vi "LabVIEW_Example.vi"() -> ()   [LabVIEW 2016]
panel:
  in  "stop":bool
  in  "Tab Control":enum32{"Navigation", "Interface", "About"}(tab)
  out "MoveSignal":bool caption="Moving"
  out "Connected":bool=TRUE
  out "EotrightDetected1":bool caption="Status Eot FWD"
  out "EotLeftDetected1":bool caption="Status Eot BWD"
  out "move out":bool=TRUE caption="Move"
  out "in target range1":bool
  in  "Reset Error":bool
  out "Error":bool
  out "Error Message":string
  in  "Axis Tab Control":enum32{"Operation", "Settings"}(tab)
  out "R [Ohm]":dbl
  out "C [nF]":dbl
  in  "Single Step\nLeft":bool caption="Open Loop Funktions"
  in  "Single Step\nRight":bool caption="Step(s)"
  in  "Continuous Forward 2":bool caption="Continuous\nForward"
  in  "Endless Left":bool caption="Continuous\nBackward"
  in  "Amplitude [V]":dbl=45.001 format="%#.3f"
  in  "Frequency [Hz]":dbl=1998.531 format="%#.3f"
  in  "Fixed DC 1":i32 caption="DC Level [mV]"
  in  "Axis 1":bool caption="Closed Loop Functions"
  out "Position":dbl=14701.126 caption="Position [nm]" format="%#_6f"
  out "Reference":dbl=-7597148.0 caption="Reference position [nm]" format="%#_6f"
  out "ReferenceSignal":bool=TRUE
  in  "measureC&R":bool
  in  "Target Position 1":i32 caption="Target position [µm]"
  in  "Move 2":bool
  in  "Positioner":u16(ring)=15 items=["ECGp5050", "ECGt5050", "ECR3030", "ECR4040", "ECR5050", "ECSx3030", "ECSx3040", "ECSx3050", "ECSx3060", "ECSx3070", "ECSx3080", "ECSx5050", "ECSxy5050", "ECSz3030", "ECSz5050", "EOP1", "EOP2", "EOP3"]
  in  "Number of steps":i32=1 caption="Number of Steps"
  in  "stop_on_EoT":bool caption="Stop on end of travel"
  in  "Target Range 1":u32 caption="Target Range [nm]"
  in  "Sensor Settings Tab Control":enum32{"NUM only", "RES only"}(tab)
  in  "auto Reset 1":bool=TRUE caption="Auto Reset"
  in  "Reference Auto Update 1":bool=TRUE caption="Auto update reference"
  in  "Configuration upload":path
  in  "Gound on target":bool
  in  "Sensor power":enum16{"0 dB", "-10 dB", "-15 dB", "-20 dB"}(ring)
  out "LutSN":string
  in  "auto measure C and R":bool
  in  "Disable Sensor":bool
  in  "Motion control threshold [pm]":i32
  in  "Output":bool=TRUE caption="Axis 1"
  out "Output Status":bool=TRUE
  out "status":string
  out "RT Out Tab Control":enum32{"Off", "AquadB", "Trigger"}(tab)
  in  "AqaudB clock 1":i32 caption="AquadB Clock\n[ns], multiple of 40ns"
  in  "AquadB Resolution 1":i32 caption="AquadB\nResolution [nm]"
  in  "Trigger Config":T1
  out "Error 4":bool caption="Error"
  out "Error Message 4":string
  in  "Mode Input":u16(ring) caption="Mode" items=["Trigger (LVDS)"=11, "Trigger (LVTTL)"=10, "Stepper (LVDS)"=9, "Stepper (LVTTL)"=8, "AquadB (LVDS)"=1, "AquadB (LVTTL)"=0, "OFF"=15]
  in  "Loop Mode":u16(ring) caption="Loop mode" items=["closed-loop"=1, "open-loop"=0]
  in  "Steps per pulse":i32 caption="Steps per pulse [Steps]"
  in  "Change per pulse":i32 caption="Change per pulse [u°/nm]"
  in  "Reset Error 4":bool
  in  "Move":bool=TRUE
  in  "Signal mode":enum16{"LVTTL", "LVDS"}(ring)
  in  "RtOutMode":enum16{"Off", "AquadB", "Trigger"}(ring)
  in  "Reboot":bool
  in  "Factory Reset":bool
  in  "Reset Error 8":bool
  out "Error Message 7":string
  in  "device name (set)":string="myAMC300" caption="Set Device Name"
  out "Error 7":bool caption="Error"
  out "Sn":string caption="Serial Number"
  out "ip":string="192.168.1.1" caption="IP Adress"
  out "Firmware Version":string
  out "Mac Adress":string
  out "authorized\nStatus":bool
  out "locked\nStatus":bool
  out "device name":string caption="Device Name"
  out "Device type":string="AMC100/NUM"
  in  "Unlock":bool=TRUE
  out "Features acivated":string[](array[string])
  in  "Lock":bool=TRUE
  in  "grant access":bool=TRUE
  # "Individual Status Flags"
  # "Closed Loop Functions"
  # "(NUM only)"
  # "Diagnostic Tools (AMC300 only)"
  # "( /PRO Version only )"
  # "( /PRO Version only )"
  # "(AMC300 only)"
  # "Real Time Input"
  # "Real Time Output"
  # "Global Parameters"
  # "Axis 1"
  # "Axis 1"
  # "Device Info"
  # "Device Access"
  # "Features activated"
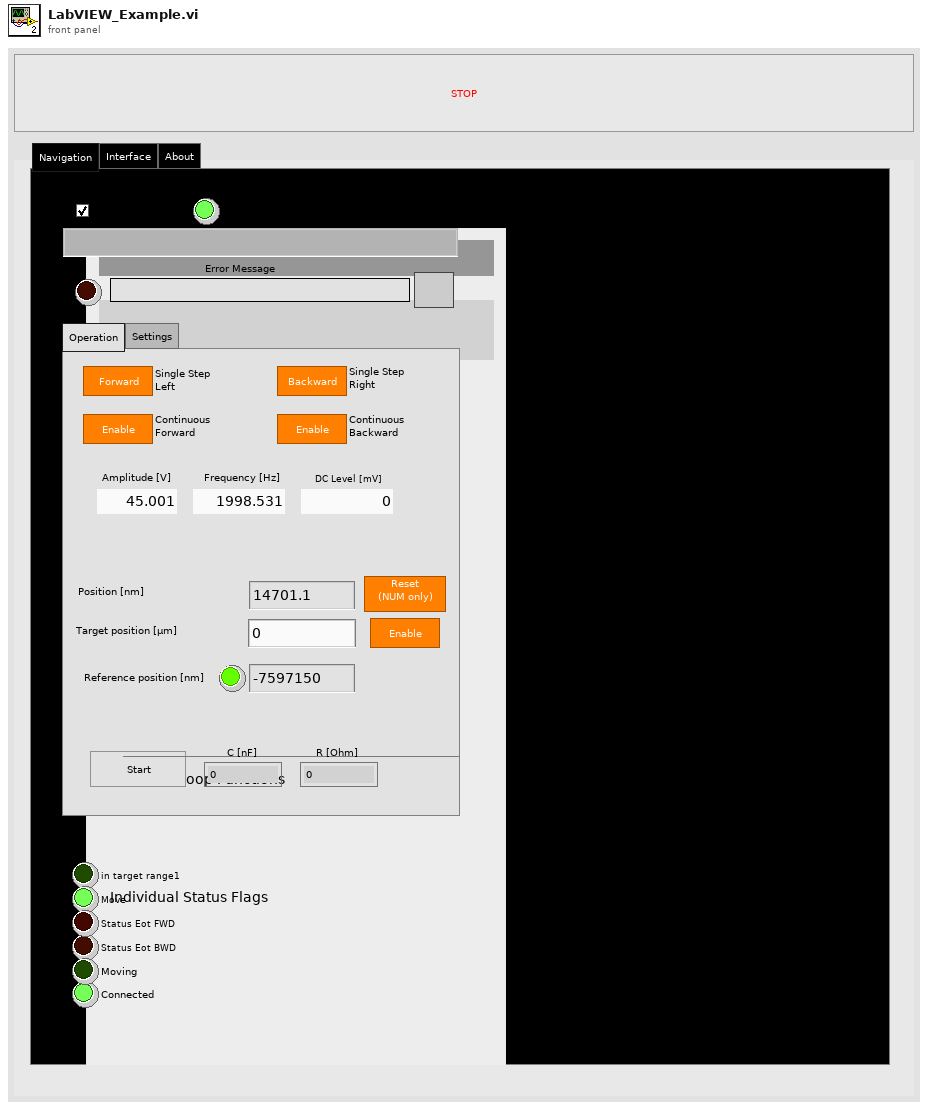
[diagram p1: front panel]
types:
  T1 = cluster{"Position high [nm]":i32, "Position low [nm]":i32, "Trigger polarity":enum16{"Active high", "Active low"}, "Epsilon [nm]":i32}
  T2 = enum8{"Enabled", "Disabled", "Disabled and Grayed Out"}
  T3 = cluster{"serial number":string, "IP address":string, "device type":string, "mac address":string, "device name":string, "firmware version":string}
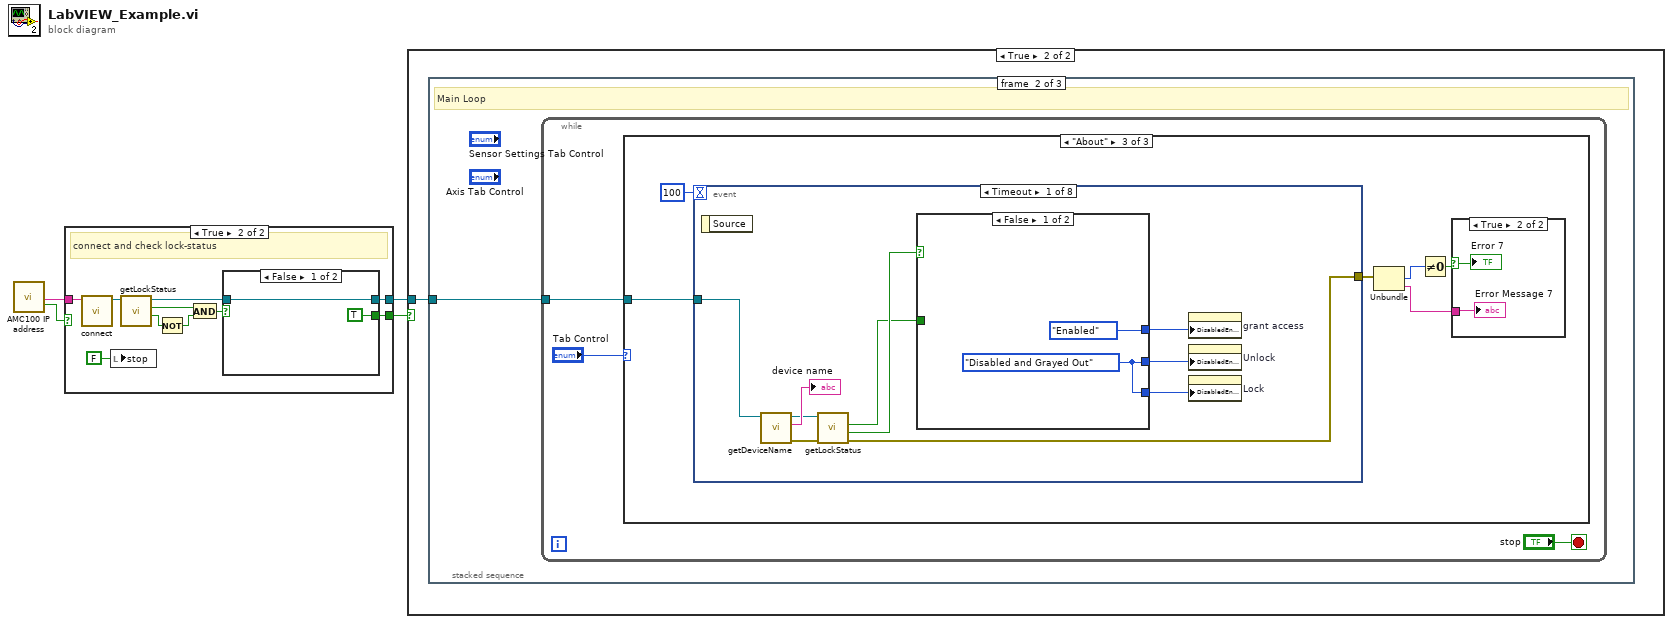
[diagram p0: block diagram]
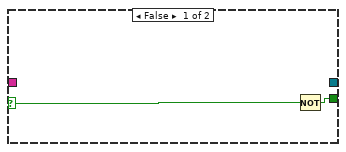
[diagram p2: hidden frame]
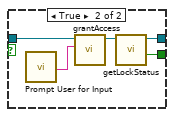
[diagram p3: hidden frame]
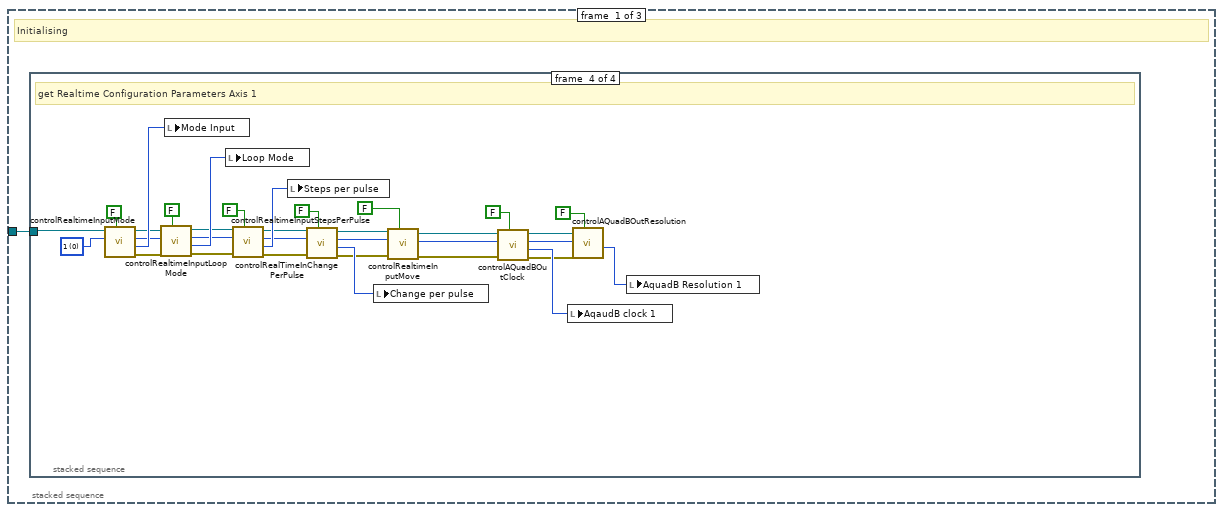
[diagram p5: hidden frame]
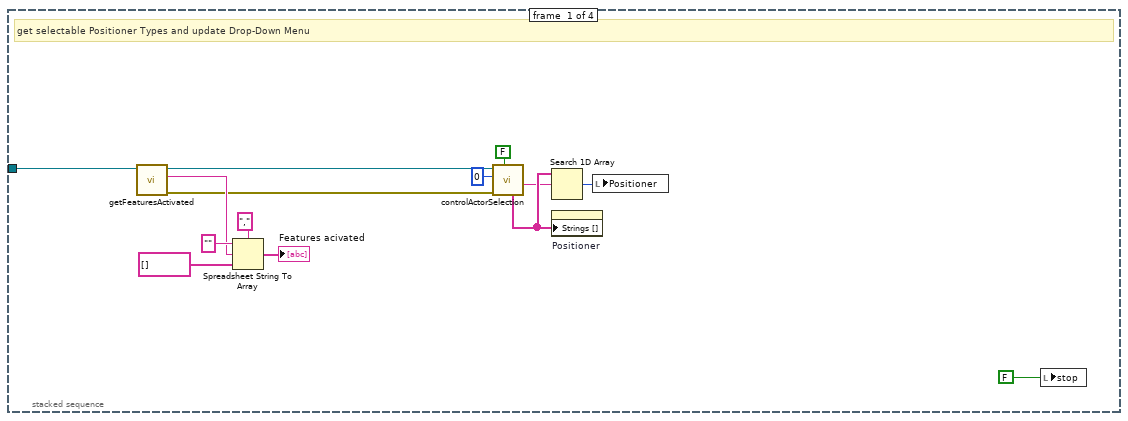
[diagram p6: hidden frame]
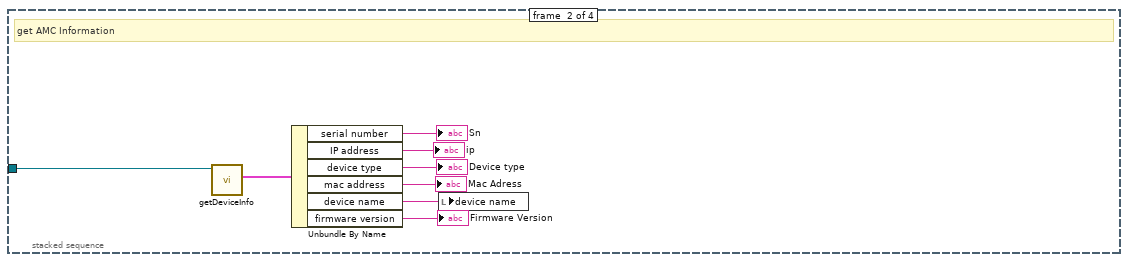
[diagram p7: hidden frame]
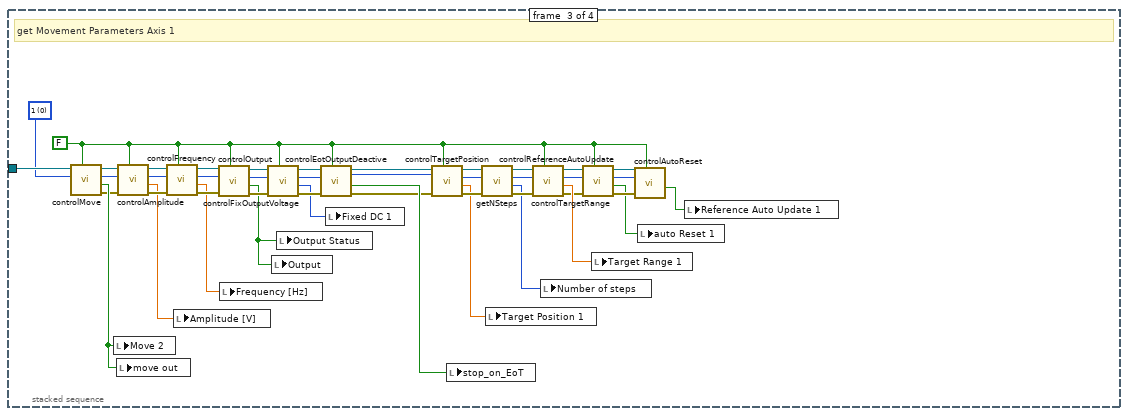
[diagram p8: hidden frame]
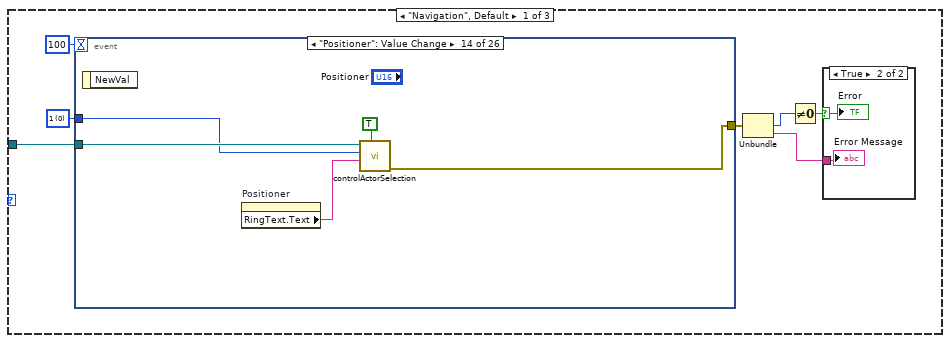
[diagram p9: hidden frame]
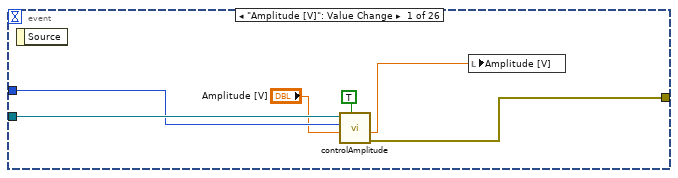
[diagram p11: hidden frame]
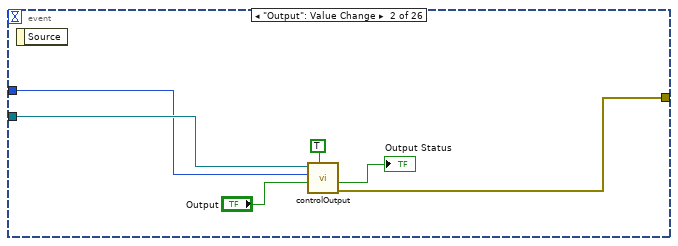
[diagram p12: hidden frame]
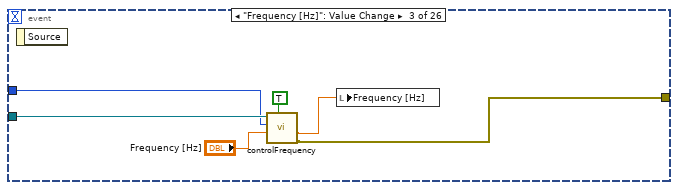
[diagram p13: hidden frame]
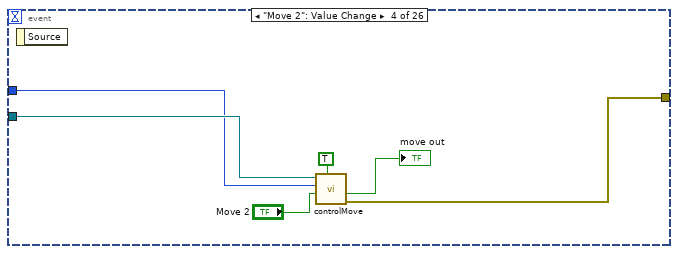
[diagram p14: hidden frame]
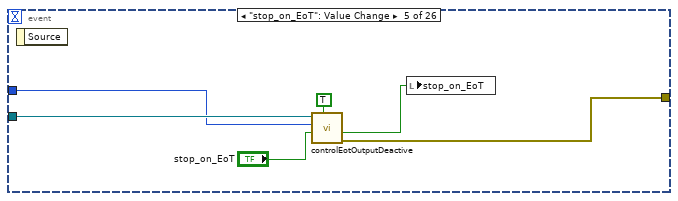
[diagram p15: hidden frame]
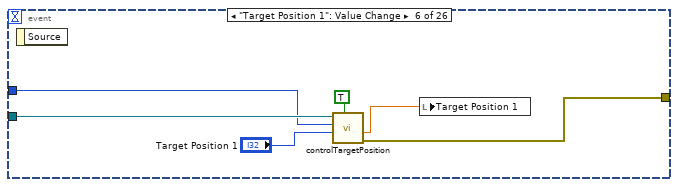
[diagram p16: hidden frame]
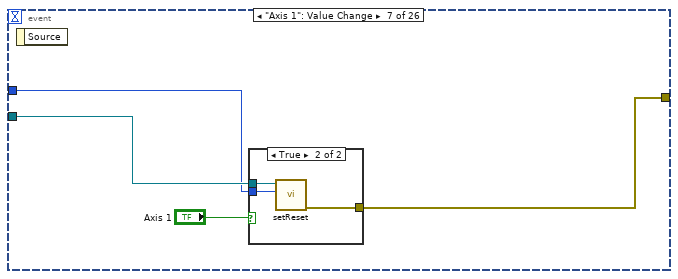
[diagram p17: hidden frame]
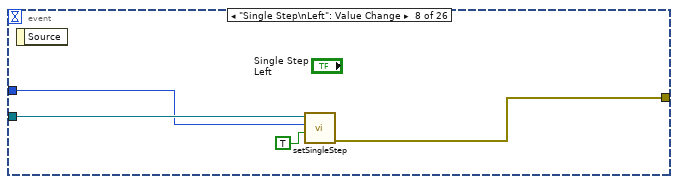
[diagram p19: hidden frame]
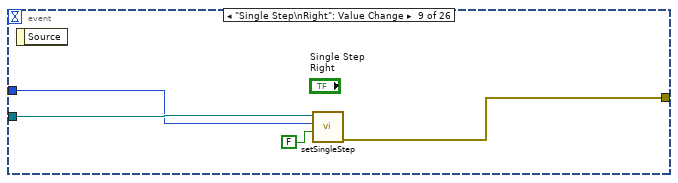
[diagram p20: hidden frame]
diagram:
  n1 = call "AMC100 IP address"() -> ("IP address"=w1:string, "OK"=w2:bool)  [unwired: 17 in, 1 out]
  n2 = case shown="True" w2 {
    selector: w2 -> [w5 _]
    tunnel: [w6 w16] -> w4
    tunnel: [_ w15] -> w3
    tunnel: w1 -> [_ w9]
    frame False {
      n3 = Not(x=w5) -> (.not. x?=w6:bool)
    }
    frame True {
      # "connect and check lock-status"
      n4 = call "connect.vi"("deviceAddress"=w9) -> ("connection ID"=w8:refnum<k5>)  [unwired: 5 in, 1 out]
      n5 = local write "stop"(FALSE ("stop")) -> ()
      n6 = call "getLockStatus.vi"("connection ID"=w8) -> ("authorized"=w11:bool, "locked"=w12:bool, "connection ID"=w14:refnum<k5>)  [unwired: 7 in, 1 out]
      n7 = Not(x=w11) -> (.not. x?=w10:bool)
      n8 = And(x=w12, y=w10) -> (x .and. y?=w13:bool)
      n9 = case shown="False" w13 {
        tunnel: w14 -> [w18 w23]
        tunnel: [w18 w20] -> w15
        tunnel: [TRUE ("authorized") w19] -> w16
        frame False {
        }
        frame True {
          n10 = call "Prompt User for Input"() -> ("password"=w22:string)  [unwired: 17 in, 2 out]
          n11 = call "grantAccess.vi"("password"=w22, "connection ID"=w23) -> ("connection ID"=w21:refnum<k5>)  [unwired: 8 in, 1 out]
          n12 = call "getLockStatus.vi"("connection ID"=w21) -> ("authorized"=w19:bool, "connection ID"=w20:refnum<k5>)  [unwired: 7 in, 2 out]
        }
      }
    }
  }
  n13 = case shown="True" w4 {
    tunnel: w3 -> [_ w24]
    frame False {
    }
    frame True {
      n14 = stacked-sequence {
        tunnel: w24 -> [w25 w125 w539]
        frame #0 {
          # "Initialising"
          n15 = stacked-sequence {
            tunnel: w25 -> [w37 w40 w57 w124]
            frame #0 {
              # "get selectable Positioner Types and update Drop-Down Menu"
              n16 = call "getFeaturesActivated.vi"("connection ID"=w37) -> ("error out"=w31:errorcluster, "features"=w34:string, "connection ID"=w26:refnum<k5>)  [unwired: 8 in]
              n17 = Spreadsheet String To Array(delimiter (Tab)=",", format string="", spreadsheet string=w34, array type (2D Dbl)=string[] []) -> (array=→"Features acivated":string[])
              n18 = call "controlActorSelection.vi"("set"=FALSE, "error in"=w31, "axis"=u8 0 ("axis in"), "connection ID"=w26) -> ("Positioner out"=w27:string, "allPositioners"=w30:string[])  [unwired: 3 in, 3 out]
              n19 = Search 1D Array(1D array=w30, element=w27) -> (index of element=w38:i32)  [unwired: 1 in]
              n20 = property on="Positioner" class="Ring (strict)"("Strings []"=w30) -> ()  [unwired: 2 in, 2 out]
              n21 = local write "Positioner"(w38) -> ()
              n22 = local write "stop"(FALSE ("stop")) -> ()
            }
            frame #1 {
              # "get AMC Information"
              n23 = call "getDeviceInfo.vi"("connection ID in"=w40) -> ("device info"=w47:T3)  [unwired: 8 in, 2 out]
              n24 = Unbundle By Name(w47) -> ("serial number"=→"Sn":string, "IP address"=→"ip":string, "device type"=→"Device type":string, "mac address"=→"Mac Adress":string, "device name"=w42:string, "firmware version"=→"Firmware Version":string)
              n25 = local write "device name"(w42) -> ()
            }
            frame #2 {
              w55 = u8 0 items=["1", "2", "3"] ("axis")
              w58 = FALSE ("set")
              # "get Movement Parameters Axis 1"
              n26 = call "controlMove.vi"("Set"=w58, "axis in"=w55, "connection ID"=w57) -> ("error out"=w52:errorcluster, "controll move out"=w53:bool, "axis out"=w54:u8, "connection ID"=w56:refnum<k5>)  [unwired: 5 in]
              n27 = local write "Move 2"(w53) -> ()
              n28 = local write "move out"(w53) -> ()
              n29 = call "controlAmplitude.vi"("Set"=w58, "error in"=w52, "axis in"=w54, "connection ID"=w56) -> ("error out"=w89:errorcluster, "amplitude [V] out"=w73:dbl, "axis out"=w91:i32, "connection ID"=w90:refnum<k5>)  [unwired: 4 in]
              n30 = call "controlFrequency.vi"("Set"=w58, "error in"=w89, "axis in"=w91, "connection ID"=w90) -> ("error out"=w86:errorcluster, "Frequenzy [Hz] out"=w72:dbl, "axis out"=w87:u8, "connection ID"=w88:refnum<k5>)  [unwired: 4 in]
              n31 = local write "Amplitude [V]"(w73) -> ()
              n32 = call "controlOutput.vi"("Set"=w58, "error in"=w86, "axis in"=w87, "connection ID"=w88) -> ("error out"=w83:errorcluster, "enable output out"=w51:bool, "axis out"=w84:u8, "connection ID"=w85:refnum<k5>)  [unwired: 4 in]
              n33 = local write "Frequency [Hz]"(w72) -> ()
              n34 = call "controlFixOutputVoltage.vi"("set"=w58, "error in"=w83, "axis in"=w84, "connection ID"=w85) -> ("error out"=w80:errorcluster, "Fixed Output Voltage in mV out"=w71:i32, "axis out"=w81:u8, "connection ID"=w82:refnum<k5>)  [unwired: 4 in]
              n35 = local write "Output"(w51) -> ()
              n36 = local write "Output Status"(w51) -> ()
              n37 = call "controlEotOutputDeactive.vi"("Set"=w58, "error in"=w80, "axis in"=w81, "connection ID"=w82) -> ("error out"=w48:errorcluster, "enable EOT out"=w70:bool, "axis out"=w49:u8, "connection ID"=w50:refnum<k5>)  [unwired: 4 in]
              n38 = local write "Fixed DC 1"(w71) -> ()
              n39 = call "controlTargetPosition.vi"("Set"=w58, "error in"=w48, "axis in"=w49, "connection ID"=w50) -> ("error out"=w77:errorcluster, "Target Position out"=w69:dbl, "axis out"=w78:u8, "connection ID"=w79:refnum<k5>)  [unwired: 4 in]
              n40 = local write "stop_on_EoT"(w70) -> ()
              n41 = call "getNSteps.vi"("error in"=w77, "axis"=w78, "connection ID"=w79) -> ("error out"=w74:errorcluster, "nbrstep"=w68:i32, "axis_out"=w75:i32, "connection ID"=w76:refnum<k5>)  [unwired: 5 in]
              n42 = local write "Target Position 1"(w69) -> ()
              n43 = call "controlTargetRange.vi"("Set"=w58, "error in"=w74, "axis in"=w75, "connection ID"=w76) -> ("error out"=w64:errorcluster, "Target Range out"=w67:dbl, "axis out"=w65:u8, "connection ID"=w66:refnum<k5>)  [unwired: 4 in]
              n44 = local write "Number of steps"(w68) -> ()
              n45 = call "controlReferenceAutoUpdate.vi"("Set"=w58, "error in"=w64, "axis in"=w65, "connection ID"=w66) -> ("error out"=w61:errorcluster, "ref auto up out"=w60:bool, "axis out"=w62:u8, "connection ID"=w63:refnum<k5>)  [unwired: 4 in]
              n46 = local write "Target Range 1"(w67) -> ()
              n47 = call "controlAutoReset.vi"("Set"=w58, "error in"=w61, "axis in"=w62, "connection ID"=w63) -> ("auto reset out"=w59:bool)  [unwired: 4 in, 3 out]
              n48 = local write "auto Reset 1"(w60) -> ()
              n49 = local write "Reference Auto Update 1"(w59) -> ()
            }
            frame #3 {
              w96 = u8 0 items=["1", "2", "3"] ("axis")
              # "get Realtime Configuration Parameters Axis 1"
              n50 = call "controlRealtimeInputMode.vi"("Set"=FALSE, "axis in"=w96, "connection ID"=w124) -> ("error out"=w107:errorcluster, "RT Mode out"=w123:i32, "axis out"=w102:u8, "connection ID"=w97:refnum<k5>)  [unwired: 5 in]
              n51 = call "controlRealtimeInputLoopMode.vi"("Set"=FALSE, "error in"=w107, "axis in"=w102, "connection ID"=w97) -> ("error out"=w108:errorcluster, "RT Loop out"=w122:i32, "axis out"=w103:u8, "connection ID"=w98:refnum<k5>)  [unwired: 4 in]
              n52 = local write "Mode Input"(w123) -> ()
              n53 = local write "Loop Mode"(w122) -> ()
              n54 = call "controlRealtimeInputStepsPerPulse.vi"("Set"=FALSE, "error in"=w108, "axis in"=w103, "connection ID"=w98) -> ("error out"=w109:errorcluster, "Steps out"=w121:i32, "axis out"=w104:u8, "connection ID"=w99:refnum<k5>)  [unwired: 4 in]
              n55 = local write "Steps per pulse"(w121) -> ()
              n56 = call "controlRealTimeInChangePerPulse.vi"("Set"=FALSE, "error in"=w109, "axis in"=w104, "connection ID"=w99) -> ("error out"=w110:errorcluster, "Change out"=w120:i32, "axis out"=w105:u8, "connection ID"=w100:refnum<k5>)  [unwired: 4 in]
              n57 = local write "Change per pulse"(w120) -> ()
              n58 = call "controlRealtimeInputMove.vi"("Set"=FALSE, "error in"=w110, "axis in"=w105, "connection ID"=w100) -> ("error out"=w92:errorcluster, "axis out"=w93:u8, "connection ID"=w94:refnum<k5>)  [unwired: 4 in, 1 out]
              n59 = call "controlAQuadBOutClock.vi"("Set"=FALSE, "error in"=w92, "axis in"=w93, "connection ID"=w94) -> ("error out"=w111:errorcluster, "clock out"=w119:i32, "axis out"=w106:u8, "connection ID"=w101:refnum<k5>)  [unwired: 4 in]
              n60 = local write "AqaudB clock 1"(w119) -> ()
              n61 = call "controlAQuadBOutResolution.vi"("Set"=FALSE, "error in"=w111, "axis in"=w106, "connection ID"=w101) -> ("ABoutRes out"=w118:i32)  [unwired: 4 in, 3 out]
              n62 = local write "AquadB Resolution 1"(w118) -> ()
            }
          }
        }
        frame #1 {
          # "Main Loop"
          n63 = while {
            tunnel: w125 -> [w126]
            stop <- "stop" stop-if-true
            n64 = case shown="\"About\"" "Tab Control" {
              tunnel: w126 -> [w135 w353 w494]
              frame "Navigation", Default {
                w134 = u8 0 items=["1", "2", "3"] ("axis in")
                n65 = event shown="[13] \"Positioner\": Value Change" {
                  selector: _ -> [_ _ _ _ _ _ _ _ _ _ _ _ _ _ _ _ _ _ _ _ _ _ _ _ _ _]
                  dyn-events: _ -> [_ _ _ _ _ _ _ _ _ _ _ _ _ _ _ _ _ _ _ _ _ _ _ _ _ _]
                  timeout: 100 -> [_ _ _ _ _ _ _ _ _ _ _ _ _ _ _ _ _ _ _ _ _ _ _ _ _ _]
                  tunnel: w134 -> [w141 w147 w152 w159 w165 w171 w176 w182 w187 w191 w202 w214 _ w222 w227 w233 w238 w243 w250 w259 w267 w273 w282 w285 w291 w305]
                  tunnel: [w139 w144 w151 w156 w163 w169 w174 w181 w185 w189 w200 w211 _ w220 w225 w231 w237 w242 w246 w257 w262 w271 w277 w284 w289 w298] -> w129
                  tunnel: w135 -> [w142 w148 w154 w160 w166 w172 w177 w183 w188 w192 w203 w215 _ w223 w228 w234 w240 w244 w251 w260 w268 w274 w283 w287 w292 w327]
                  event "Amplitude [V]": Value Change {
                    n66 = event-data() -> ()  [unwired: 1 in, 1 out]
                    n67 = call "controlAmplitude.vi"("Set"=TRUE, "amplitude [V] in"="Amplitude [V]", "axis in"=w141, "connection ID"=w142) -> ("error out"=w139:errorcluster, "amplitude [V] out"=w138:dbl)  [unwired: 4 in, 2 out]
                    n68 = local write "Amplitude [V]"(w138) -> ()
                  }
                  event "Output": Value Change {
                    n69 = event-data() -> ()  [unwired: 1 in, 1 out]
                    n70 = call "controlOutput.vi"("Set"=TRUE, "enable output in"="Output", "axis in"=w147, "connection ID"=w148) -> ("error out"=w144:errorcluster, "enable output out"=→"Output Status":bool)  [unwired: 4 in, 2 out]
                  }
                  event "Frequency [Hz]": Value Change {
                    n71 = event-data() -> ()  [unwired: 1 in, 1 out]
                    n72 = call "controlFrequency.vi"("Set"=TRUE, "Frequenzy [Hz] in"="Frequency [Hz]", "axis in"=w152, "connection ID"=w154) -> ("error out"=w151:errorcluster, "Frequenzy [Hz] out"=w150:dbl)  [unwired: 4 in, 2 out]
                    n73 = local write "Frequency [Hz]"(w150) -> ()
                  }
                  event "Move 2": Value Change {
                    n74 = event-data() -> ()  [unwired: 1 in, 1 out]
                    n75 = call "controlMove.vi"("Set"=TRUE, "control move in"="Move 2", "axis in"=w159, "connection ID"=w160) -> ("error out"=w156:errorcluster, "controll move out"=→"move out":bool)  [unwired: 4 in, 2 out]
                  }
                  event "stop_on_EoT": Value Change {
                    n76 = event-data() -> ()  [unwired: 1 in, 1 out]
                    n77 = call "controlEotOutputDeactive.vi"("Set"=TRUE, "enable EOT in"="stop_on_EoT", "axis in"=w165, "connection ID"=w166) -> ("error out"=w163:errorcluster, "enable EOT out"=w162:bool)  [unwired: 4 in, 2 out]
                    n78 = local write "stop_on_EoT"(w162) -> ()
                  }
                  event "Target Position 1": Value Change {
                    n79 = event-data() -> ()  [unwired: 1 in, 1 out]
                    n80 = call "controlTargetPosition.vi"("Set"=TRUE, "Target Position in"="Target Position 1", "axis in"=w171, "connection ID"=w172) -> ("error out"=w169:errorcluster, "Target Position out"=w168:dbl)  [unwired: 4 in, 2 out]
                    n81 = local write "Target Position 1"(w168) -> ()
                  }
                  event "Axis 1": Value Change {
                    n82 = event-data() -> ()  [unwired: 1 in, 1 out]
                    n83 = case shown="True" "Axis 1" {
                      tunnel: [_ w180] -> w174
                      tunnel: w177 -> [_ w179]
                      tunnel: w176 -> [_ w178]
                      frame False {
                      }
                      frame True {
                        n84 = call "setReset.vi"("axis"=w178, "connection ID"=w179) -> ("error out"=w180:errorcluster)  [unwired: 7 in, 2 out]
                      }
                    }
                  }
                  event "Single Step\nLeft": Value Change {
                    n85 = event-data() -> ()  [unwired: 1 in, 1 out]
                    n86 = call "setSingleStep.vi"("backward"=TRUE ("FWD"), "axis"=w182, "connection ID"=w183) -> ("error out"=w181:errorcluster)  [unwired: 6 in, 2 out]
                  }
                  event "Single Step\nRight": Value Change {
                    n87 = event-data() -> ()  [unwired: 1 in, 1 out]
                    n88 = call "setSingleStep.vi"("backward"=FALSE ("FWD"), "axis"=w187, "connection ID"=w188) -> ("error out"=w185:errorcluster)  [unwired: 6 in, 2 out]
                  }
                  event "Endless Left": Value Change {
                    n89 = event-data() -> ()  [unwired: 1 in, 1 out]
                    n90 = call "controlContinousFwd.vi"("Set"=TRUE, "continous FWD in"=FALSE, "axis in"=w191, "connection ID"=w192) -> ("error out"=w193:errorcluster, "axis out"=w197:u8, "connection ID"=w198:refnum<k5>)  [unwired: 4 in, 1 out]
                    n91 = call "controlContinousBkwd.vi"("Set"=TRUE, "error in"=w193, "continous BWD in"="Endless Left", "axis in"=w197, "connection ID"=w198) -> ("error out"=w189:errorcluster)  [unwired: 3 in, 3 out]
                    n92 = local write "Continuous Forward 2"(FALSE) -> ()
                  }
                  event "Continuous Forward 2": Value Change {
                    n93 = event-data() -> ()  [unwired: 1 in, 1 out]
                    n94 = call "controlContinousBkwd.vi"("Set"=TRUE, "continous BWD in"=FALSE, "axis in"=w202, "connection ID"=w203) -> ("error out"=w204:errorcluster, "axis out"=w208:u8, "connection ID"=w209:refnum<k5>)  [unwired: 4 in, 1 out]
                    n95 = call "controlContinousFwd.vi"("Set"=TRUE, "error in"=w204, "continous FWD in"="Continuous Forward 2", "axis in"=w208, "connection ID"=w209) -> ("error out"=w200:errorcluster)  [unwired: 3 in, 3 out]
                    n96 = local write "Endless Left"(FALSE) -> ()
                  }
                  event "Fixed DC 1": Value Change {
                    n97 = event-data() -> ()  [unwired: 1 in, 1 out]
                    n98 = call "controlFixOutputVoltage.vi"("set"=TRUE ("Set"), "Fixed Output Voltage in mV"="Fixed DC 1", "axis in"=w214, "connection ID"=w215) -> ("error out"=w211:errorcluster, "Fixed Output Voltage in mV out"=w212:i32)  [unwired: 4 in, 2 out]
                    n99 = local write "Fixed DC 1"(w212) -> ()
                  }
                  event "Reset Error": Value Change {
                    n100 = event-data() -> ()  [unwired: 1 in, 1 out]
                    n101 = local write "Error Message"("" ("Error Message")) -> ()
                    n102 = local write "Error"(FALSE ("Error")) -> ()
                  }
                  event "Positioner": Value Change {
                    n103 = event-data() -> ()  [unwired: 1 in, 1 out]
                    n104 = property on="Positioner" class="Ring (strict)"() -> ("RingText.Text"=w221:string)  [unwired: 2 in, 2 out]
                    n105 = call "controlActorSelection.vi"("set"=TRUE, "Positioner in"=w221, "axis"=w222, "connection ID"=w223) -> ("error out"=w220:errorcluster)  [unwired: 3 in, 4 out]
                  }
                  event "Target Range 1": Value Change {
                    n106 = event-data() -> ()  [unwired: 1 in, 1 out]
                    n107 = call "controlTargetRange.vi"("Set"=TRUE, "Target Range in"="Target Range 1", "axis in"=w227, "connection ID"=w228) -> ("error out"=w225:errorcluster, "Target Range out"=w224:dbl)  [unwired: 4 in, 2 out]
                    n108 = local write "Target Range 1"(w224) -> ()
                  }
                  event "auto Reset 1": Value Change {
                    n109 = event-data() -> ()  [unwired: 1 in, 1 out]
                    n110 = call "controlAutoReset.vi"("Set"=TRUE, "auto reset in"="auto Reset 1", "axis in"=w233, "connection ID"=w234) -> ("error out"=w231:errorcluster, "auto reset out"=w230:bool)  [unwired: 4 in, 2 out]
                    n111 = local write "auto Reset 1"(w230) -> ()
                  }
                  event "Reference Auto Update 1": Value Change {
                    n112 = event-data() -> ()  [unwired: 1 in, 1 out]
                    n113 = call "controlReferenceAutoUpdate.vi"("Set"=TRUE, "ref auto up in"="Reference Auto Update 1", "axis in"=w238, "connection ID"=w240) -> ("error out"=w237:errorcluster, "ref auto up out"=w236:bool)  [unwired: 4 in, 2 out]
                    n114 = local write "Reference Auto Update 1"(w236) -> ()
                  }
                  event "Configuration upload": Value Change {
                    n115 = event-data() -> ()  [unwired: 1 in, 1 out]
                    n116 = call "loadLutFile.vi"("connection ID"=w244, "axis"=w243, "Path to LUT file"="Configuration upload") -> ("error out"=w242:errorcluster)  [unwired: 10 in, 2 out]
                  }
                  event "measureC&R": Value Change {
                    n117 = event-data() -> ()  [unwired: 1 in, 1 out]
                    n118 = call "measureCapacitanceAndResistance.vi"("axis"=w250, "connection ID in"=w251) -> ("error out"=w246:errorcluster, "results"=w249:cluster{"capacitance":dbl, "resistance":dbl})  [unwired: 6 in, 2 out]
                    n119 = case shown="No Error" w246 {
                      tunnel: w249 -> [w254 _]
                      tunnel: [w253 w255] -> w248
                      tunnel: [w252 w255] -> w247
                      frame No Error {
                        n120 = Unbundle By Name(w254) -> ("capacitance"=w253:dbl, "resistance"=w252:dbl)
                      }
                      frame Error {
                        w255 = nan ("capacitance")
                      }
                    }
                    "C [nF]" <- w248
                    "R [Ohm]" <- w247
                  }
                  event "Gound on target": Value Change {
                    n121 = event-data() -> ()  [unwired: 1 in, 1 out]
                    n122 = call "contolGroundAxisAutoOnTarget.vi"("Set"=TRUE, "enable"="Gound on target", "axis in"=w259, "connection ID"=w260) -> ("error out"=w257:errorcluster, "enable out"=w256:bool)  [unwired: 4 in, 2 out]
                    n123 = local write "Gound on target"(w256) -> ()
                  }
                  event "auto measure C and R": Value Change {
                    n124 = event-data() -> ()  [unwired: 1 in, 1 out]
                    n125 = call "setAutoMeasure.vi"("enable"="auto measure C and R", "axis"=w267, "connection ID"=w268) -> ("error out"=w266:errorcluster, "axis_out"=w264:i32, "connection ID"=w265:refnum<k5>)  [unwired: 6 in]
                    n126 = call "getAutoMeasure.vi"("error in"=w266, "axis"=w264, "connection ID"=w265) -> ("error out"=w262:errorcluster, "enable"=w263:bool)  [unwired: 5 in, 2 out]
                    n127 = local write "auto measure C and R"(w263) -> ()
                  }
                  event "Sensor power": Value Change {
                    n128 = event-data() -> ()  [unwired: 1 in, 1 out]
                    n129 = call "controlChainGain.vi"("Set"=TRUE, "gainconfig"="Sensor power", "axis in"=w273, "connection ID"=w274) -> ("error out"=w271:errorcluster, "gainconfig out"=w270:enum16{"0 dB", "-10 dB", "-15 dB", "-20 dB"})  [unwired: 4 in, 2 out]
                    n130 = local write "Sensor power"(w270) -> ()
                  }
                  event "Disable Sensor": Value Change {
                    n131 = event-data() -> ()  [unwired: 1 in, 1 out]
                    n132 = Not(x="Disable Sensor") -> (.not. x?=w279:bool)
                    n133 = call "controlSensorEnabled.vi"("set"=TRUE, "enableSensor"=w279, "axis"=w282, "connection ID"=w283) -> ("error out"=w277:errorcluster, "enableSensor out"=w276:bool)  [unwired: 4 in, 2 out]
                    n134 = Not(x=w276) -> (.not. x?=w278:bool)
                    n135 = local write "Disable Sensor"(w278) -> ()
                  }
                  event "Number of steps": Value Change {
                    n136 = event-data() -> ()  [unwired: 1 in, 1 out]
                    n137 = call "writeNSteps.vi"("step"="Number of steps", "axis"=w285, "connection ID"=w287) -> ("error out"=w284:errorcluster)  [unwired: 6 in, 2 out]
                  }
                  event "Motion control threshold [pm]": Value Change {
                    n138 = event-data() -> ()  [unwired: 1 in, 1 out]
                    n139 = call "controlMotionControlThreshold.vi"("Set"=TRUE, "threshold"="Motion control threshold [pm]", "axis in"=w291, "connection ID"=w292) -> ("error out"=w289:errorcluster, "threshold out"=w288:i32)  [unwired: 4 in, 2 out]
                    n140 = local write "Motion control threshold [pm]"(w288) -> ()
                  }
                  event Timeout {
                    n141 = event-data() -> ()  [unwired: 1 in, 1 out]
                    n142 = call "getPosition.vi"("axis"=w305, "connection ID"=w327) -> ("error out"=w320:errorcluster, "position"=→"Position":dbl, "axis_out"=w340:i32, "connection ID"=w341:refnum<k5>)  [unwired: 6 in]
                    n143 = call "getReferencePosition.vi"("error in"=w320, "axis"=w340, "connection ID"=w341) -> ("error out"=w319:errorcluster, "position"=→"Reference":i32, "axis_out"=w338:i32, "connection ID"=w339:refnum<k5>)  [unwired: 5 in]
                    n144 = call "getStatusConnected.vi"("error in"=w319, "axis"=w338, "connection ID"=w339) -> ("error out"=w318:errorcluster, "connected"=→"Connected":bool, "axis_out"=w336:i32, "connection ID"=w337:refnum<k5>)  [unwired: 5 in]
                    n145 = call "getStatusMoving.vi"("error in"=w318, "axis"=w336, "connection ID"=w337) -> ("error out"=w317:errorcluster, "status"=w302:i32, "axis_out"=w334:i32, "connection ID"=w335:refnum<k5>)  [unwired: 5 in]
                    n146 = Greater Than 0?(x=w302) -> (x > 0?=→"MoveSignal":bool)
                    n147 = call "getStatusReference.vi"("error in"=w317, "axis"=w334, "connection ID"=w335) -> ("error out"=w316:errorcluster, "valid"=→"ReferenceSignal":bool, "axis_out"=w332:i32, "connection ID"=w333:refnum<k5>)  [unwired: 5 in]
                    n148 = call "getStatusEotBkwd.vi"("error in"=w316, "axis"=w332, "connection ID"=w333) -> ("error out"=w315:errorcluster, "detected"=→"EotLeftDetected1":bool, "axis_out"=w330:i32, "connection ID"=w331:refnum<k5>)  [unwired: 5 in]
                    n149 = call "getStatusEotFwd.vi"("error in"=w315, "axis"=w330, "connection ID"=w331) -> ("error out"=w314:errorcluster, "detected"=→"EotrightDetected1":bool, "axis_out"=w328:i32, "connection ID"=w329:refnum<k5>)  [unwired: 5 in]
                    n150 = call "getStatusTargetRange.vi"("error in"=w314, "axis"=w328, "connection ID"=w329) -> ("error out"=w311:errorcluster, "in_range"=→"in target range1":bool, "axis_out"=w312:i32, "connection ID"=w313:refnum<k5>)  [unwired: 5 in]
                    n151 = call "controlMove.vi"("Set"=FALSE, "error in"=w311, "control move in"=FALSE, "axis in"=w312, "connection ID"=w313) -> ("error out"=w304:errorcluster, "controll move out"=w309:bool, "connection ID"=w306:refnum<k5>)  [unwired: 3 in, 1 out]
                    n152 = call "getFullCombinedStatus.vi"("error in"=w304, "axis"=w305, "connection ID"=w306) -> ("error out"=w294:errorcluster, "string"=→"status":string, "axis_out"=w295:i32, "connection ID"=w296:refnum<k5>)  [unwired: 5 in]
                    n153 = call "getLutSn.vi"("error in"=w294, "axis"=w295, "connection ID"=w296) -> ("error out"=w299:errorcluster, "string"=→"LutSN":string, "connection ID"=w300:refnum<k5>)  [unwired: 5 in, 1 out]
                    n154 = disable-structure shown="Disabled" {
                      disable-tunnel: w300 -> [w345 _]
                      disable-tunnel: w299 -> [w344 w346]
                      disable-tunnel: [_ w346] -> w298
                      frame Disabled {
                        n155 = call "controlLinearization.vi"("set"=FALSE, "error in"=w344, "LutUsageEnable"=FALSE, "connection ID in"=w345) -> ()  [unwired: 5 in, 3 out]
                      }
                      frame Enabled {
                      }
                    }
                    n156 = local write "move out"(w309) -> ()
                    n157 = local write "Move 2"(w309) -> ()
                  }
                }
                n158 = Unbundle(w129) -> ("code"=w131:i32, "source"=w132:string)  [unwired: 1 out]
                n159 = Not Equal To 0?(x=w131) -> (x != 0?=w130:bool)
                n160 = case shown="True" w130 {
                  selector: w130 -> [_ w136]
                  tunnel: w132 -> [_ w137]
                  frame False {
                  }
                  frame True {
                    "Error Message" <- w137
                    "Error" <- w136
                  }
                }
              }
              frame "Interface" {
                w352 = u8 0 items=["1", "2", "3"] ("axis in")
                n161 = event shown="[0] Timeout" {
                  selector: _ -> [_ _ _ _ _ _ _ _ _ _ _ _]
                  dyn-events: _ -> [_ _ _ _ _ _ _ _ _ _ _ _]
                  timeout: 100 -> [_ _ _ _ _ _ _ _ _ _ _ _]
                  tunnel: w352 -> [w359 w433 w439 w445 w451 w456 w462 w468 _ w479 w485 _]
                  tunnel: [w358 w430 w436 w441 w447 w453 w460 w466 w472 w476 w482 _] -> w349
                  tunnel: w353 -> [w360 w434 w440 w446 w452 w458 w464 w470 w474 w480 w486 _]
                  event Timeout {
                    n162 = event-data() -> ()  [unwired: 1 in, 1 out]
                    n163 = stacked-sequence {
                      tunnel: w360 -> [w373 w403]
                      tunnel: w359 -> [w372 w400]
                      tunnel: [w365 _] -> w357
                      tunnel: [_ w408] -> w356
                      frame #0 {
                        w361 = FALSE ("Set")
                        # "get RT Input\nSettings"
                        n164 = call "controlRealtimeInputStepsPerPulse.vi"("Set"=w361, "axis in"=w372, "connection ID"=w373) -> ("error out"=w368:errorcluster, "Steps out"=w374:i32, "axis out"=w364:u8, "connection ID"=w371:refnum<k5>)  [unwired: 5 in]
                        n165 = call "controlRealTimeInChangePerPulse.vi"("Set"=w361, "error in"=w368, "axis in"=w364, "connection ID"=w371) -> ("error out"=w367:errorcluster, "Change out"=w375:i32, "axis out"=w363:u8, "connection ID"=w370:refnum<k5>)  [unwired: 4 in]
                        n166 = local write "Steps per pulse"(w374) -> ()
                        n167 = call "controlRealtimeInputMove.vi"("Set"=w361, "error in"=w367, "axis in"=w363, "connection ID"=w370) -> ("error out"=w366:errorcluster, "move out"=w376:bool, "axis out"=w362:u8, "connection ID"=w369:refnum<k5>)  [unwired: 4 in]
                        n168 = local write "Change per pulse"(w375) -> ()
                        n169 = call "controlRealtimeInputMode.vi"("Set"=w361, "error in"=w366, "axis in"=w362, "connection ID"=w369) -> ("error out"=w382:errorcluster, "RT Mode out"=w385:i32, "axis out"=w383:u8, "connection ID"=w384:refnum<k5>)  [unwired: 4 in]
                        n170 = local write "Move"(w376) -> ()
                        n171 = Equal?(x=w385, y=15) -> (x = y?=w387:bool)
                        n172 = call "controlRealtimeInputLoopMode.vi"("Set"=w361, "error in"=w382, "axis in"=w383, "connection ID"=w384) -> ("error out"=w365:errorcluster, "RT Loop out"=w377:i32)  [unwired: 4 in, 2 out]
                        n173 = local write "Loop Mode"(w377) -> ()
                        n174 = local write "Mode Input"(w385) -> ()
                        n175 = Equal To 0?(x=w377) -> (x = 0?=w386:bool)
                        n176 = case shown="False" w387 {
                          tunnel: w386 -> [w393 _]
                          tunnel: [w392 w398] -> w381
                          tunnel: [w391 w398] -> w380
                          tunnel: [w390 w398] -> w379
                          tunnel: [w389 w398] -> w378
                          frame False {
                            # "RT Input ON"
                            n177 = case shown="True" w393 {
                              tunnel: [w394 w397] -> w392
                              tunnel: [w394 w396] -> w391
                              tunnel: [T2."Disabled and Grayed Out" ("Disabled") w397] -> w389
                              tunnel: [w394 w396] -> w390
                              frame False {
                                w394 = T2."Enabled" ("Disabled")
                                # "closed-loop Mode"
                              }
                              frame True {
                                w397 = T2."Enabled" ("Disabled")
                                w396 = T2."Disabled and Grayed Out" ("Disabled")
                                # "open-loop Mode"
                              }
                            }
                          }
                          frame True {
                            w398 = T2."Disabled and Grayed Out" ("Disabled")
                            # "RT Input OFF"
                          }
                        }
                        n178 = property on="Loop Mode" class="Ring (strict)"("DisabledEnum"=w381) -> ()  [unwired: 2 in, 2 out]
                        n179 = property on="Move" class="Bool (strict)"("DisabledEnum"=w379) -> ()  [unwired: 2 in, 2 out]
                        n180 = property on="Change per pulse" class="DigNum (strict)"("DisabledEnum"=w380) -> ()  [unwired: 2 in, 2 out]
                        n181 = property on="Steps per pulse" class="DigNum (strict)"("DisabledEnum"=w378) -> ()  [unwired: 2 in, 2 out]
                      }
                      frame #1 {
                        # "get RT Output\nSettings"
                        n182 = call "controlRtOutSignalMode.vi"("connection ID"=w403) -> ("error out"=w401:errorcluster, "RT out Mode out"=w407:enum16{"LVTTL", "LVDS"}, "connection ID"=w402:refnum<k5>)  [unwired: 8 in]
                        n183 = call "controlRtOutMode.vi"("set"=FALSE, "error in"=w401, "axis"=w400, "connection ID"=w402) -> ("error out"=w404:errorcluster, "RtOutMode"=w399:enum16{"Off", "AquadB", "Trigger"}, "axis_out"=w405:i32, "connection ID"=w406:refnum<k5>)  [unwired: 4 in]
                        n184 = local write "Signal mode"(w407) -> ()
                        n185 = case shown="\"Trigger\"" w399 {
                          tunnel: w406 -> [_ w418 w423]
                          tunnel: w404 -> [w410 w417 w422]
                          tunnel: w405 -> [_ w413 _]
                          tunnel: [w410 w411 w421] -> w408
                          frame "Off", Default {
                          }
                          frame "AquadB" {
                            n186 = call "controlAQuadBOutClock.vi"("error in"=w417, "axis in"=w413, "connection ID"=w418) -> ("error out"=w416:errorcluster, "clock out"=w414:i32, "axis out"=w412:u8, "connection ID"=w415:refnum<k5>)  [unwired: 5 in]
                            n187 = call "controlAQuadBOutResolution.vi"("error in"=w416, "axis in"=w412, "connection ID"=w415) -> ("error out"=w411:errorcluster, "ABoutRes out"=w419:i32)  [unwired: 5 in, 2 out]
                            n188 = local write "AqaudB clock 1"(w414) -> ()
                            n189 = local write "AquadB Resolution 1"(w419) -> ()
                          }
                          frame "Trigger" {
                            n190 = call "controlRtOutTriggerConfig.vi"("error in"=w422, "connection ID"=w423) -> ("error out"=w421:errorcluster, "Trigger Config out"=w420:T1)  [unwired: 6 in, 2 out]
                            n191 = local write "Trigger Config"(w420) -> ()
                          }
                        }
                        n192 = local write "RT Out Tab Control"(w399) -> ()
                        n193 = local write "RtOutMode"(w399) -> ()
                      }
                    }
                    n194 = Merge Errors(w357, w356) -> (w358:errorcluster)
                  }
                  event "Mode Input": Value Change {
                    n195 = event-data() -> ()  [unwired: 1 in, 1 out]
                    n196 = call "controlRealtimeInputMode.vi"("Set"=TRUE, "RT Mode in"="Mode Input", "axis in"=w433, "connection ID"=w434) -> ("error out"=w424:errorcluster, "RT Mode out"=w425:i32, "axis out"=w426:u8, "connection ID"=w427:refnum<k5>)  [unwired: 4 in]
                    n197 = local write "Mode Input"(w425) -> ()
                    n198 = call "controlRealtimeInputLoopMode.vi"("Set"=FALSE, "error in"=w424, "axis in"=w426, "connection ID"=w427) -> ("error out"=w430:errorcluster, "RT Loop out"=w429:i32)  [unwired: 4 in, 2 out]
                    n199 = local write "Loop Mode"(w429) -> ()
                  }
                  event "Loop Mode": Value Change {
                    n200 = event-data() -> ()  [unwired: 1 in, 1 out]
                    n201 = call "controlRealtimeInputLoopMode.vi"("Set"=TRUE, "RT Loop in"="Loop Mode", "axis in"=w439, "connection ID"=w440) -> ("error out"=w436:errorcluster, "RT Loop out"=w435:i32)  [unwired: 4 in, 2 out]
                    n202 = local write "Loop Mode"(w435) -> ()
                  }
                  event "Steps per pulse": Value Change {
                    n203 = event-data() -> ()  [unwired: 1 in, 1 out]
                    n204 = call "controlRealtimeInputStepsPerPulse.vi"("Set"=TRUE, "Steps in"="Steps per pulse", "axis in"=w445, "connection ID"=w446) -> ("error out"=w441:errorcluster, "Steps out"=w442:i32)  [unwired: 4 in, 2 out]
                    n205 = local write "Steps per pulse"(w442) -> ()
                  }
                  event "Change per pulse": Value Change {
                    n206 = event-data() -> ()  [unwired: 1 in, 1 out]
                    n207 = call "controlRealTimeInChangePerPulse.vi"("Set"=TRUE, "Change in"="Change per pulse", "axis in"=w451, "connection ID"=w452) -> ("error out"=w447:errorcluster, "Change out"=w448:i32)  [unwired: 4 in, 2 out]
                    n208 = local write "Change per pulse"(w448) -> ()
                  }
                  event "Move": Value Change {
                    n209 = event-data() -> ()  [unwired: 1 in, 1 out]
                    n210 = call "controlRealtimeInputMove.vi"("Set"=TRUE, "move in"="Move", "axis in"=w456, "connection ID"=w458) -> ("error out"=w453:errorcluster, "move out"=w454:bool)  [unwired: 4 in, 2 out]
                    n211 = local write "Move"(w454) -> ()
                  }
                  event "AqaudB clock 1": Value Change {
                    n212 = event-data() -> ()  [unwired: 1 in, 1 out]
                    n213 = call "controlAQuadBOutClock.vi"("Set"=TRUE, "clock in"="AqaudB clock 1", "axis in"=w462, "connection ID"=w464) -> ("error out"=w460:errorcluster, "clock out"=w459:i32)  [unwired: 4 in, 2 out]
                    n214 = local write "AqaudB clock 1"(w459) -> ()
                  }
                  event "AquadB Resolution 1": Value Change {
                    n215 = event-data() -> ()  [unwired: 1 in, 1 out]
                    n216 = call "controlAQuadBOutResolution.vi"("Set"=TRUE, "ABoutRes in"="AquadB Resolution 1", "axis in"=w468, "connection ID"=w470) -> ("error out"=w466:errorcluster, "ABoutRes out"=w465:i32)  [unwired: 4 in, 2 out]
                    n217 = local write "AquadB Resolution 1"(w465) -> ()
                  }
                  event "Signal mode": Value Change {
                    n218 = event-data() -> ()  [unwired: 1 in, 6 out]
                    n219 = call "controlRtOutSignalMode.vi"("Set"=TRUE, "RT out Mode"="Signal mode", "connection ID"=w474) -> ("error out"=w472:errorcluster, "RT out Mode out"=w471:enum16{"LVTTL", "LVDS"})  [unwired: 6 in, 1 out]
                    n220 = local write "Signal mode"(w471) -> ()
                  }
                  event "RtOutMode": Value Change {
                    n221 = event-data() -> ()  [unwired: 1 in, 1 out]
                    n222 = call "controlRtOutMode.vi"("set"=TRUE, "RtOutMode"="RtOutMode", "axis"=w479, "connection ID"=w480) -> ("error out"=w476:errorcluster, "RtOutMode"=w477:enum16{"Off", "AquadB", "Trigger"})  [unwired: 4 in, 2 out]
                    "RT Out Tab Control" <- w477
                    n223 = local write "RtOutMode"(w477) -> ()
                  }
                  event "Trigger Config": Value Change {
                    n224 = event-data() -> ()  [unwired: 1 in, 1 out]
                    n225 = call "controlRtOutTriggerConfig.vi"("Set"=TRUE, "Trigger Config"="Trigger Config", "axis in"=w485, "connection ID"=w486) -> ("error out"=w482:errorcluster, "Trigger Config out"=w483:T1)  [unwired: 4 in, 2 out]
                    n226 = local write "Trigger Config"(w483) -> ()
                  }
                  event "Reset Error 4": Value Change {
                    n227 = event-data() -> ()  [unwired: 1 in, 1 out]
                    n228 = local write "Error Message 4"("" ("Error Message")) -> ()
                    n229 = local write "Error 4"(FALSE ("Error 4")) -> ()
                  }
                }
                n230 = Unbundle(w349) -> ("code"=w347:i32, "source"=w348:string)  [unwired: 1 out]
                n231 = Not Equal To 0?(x=w347) -> (x != 0?=w350:bool)
                n232 = case shown="True" w350 {
                  selector: w350 -> [_ w354]
                  tunnel: w348 -> [_ w355]
                  frame False {
                  }
                  frame True {
                    "Error Message 4" <- w355
                    "Error 4" <- w354
                  }
                }
              }
              frame "About" {
                n233 = event shown="[0] Timeout" {
                  selector: _ -> [_ _ _ _ _ _ _ _]
                  dyn-events: _ -> [_ _ _ _ _ _ _ _]
                  timeout: 100 -> [_ _ _ _ _ _ _ _]
                  tunnel: w494 -> [w507 w523 w526 w529 w532 w534 w536 _]
                  tunnel: [w503 w522 w525 w528 w531 w533 w535 _] -> w490
                  event Timeout {
                    n234 = event-data() -> ()  [unwired: 1 in, 1 out]
                    n235 = call "getDeviceName.vi"("connection ID"=w507) -> ("error out"=w504:errorcluster, "string"=→"device name":string, "connection ID"=w505:refnum<k5>)  [unwired: 8 in]
                    n236 = call "getLockStatus.vi"("error in"=w504, "connection ID"=w505) -> ("error out"=w503:errorcluster, "authorized"=w502:bool, "locked"=w501:bool)  [unwired: 6 in, 1 out]
                    n237 = case shown="False" w502 {
                      selector: w502 -> [_ w514]
                      tunnel: w501 -> [_ w513]
                      tunnel: [T2."Enabled" ("Disabled") w512] -> w500
                      tunnel: [w509 w511] -> w499
                      tunnel: [w509 w510] -> w498
                      frame False {
                        w509 = T2."Disabled and Grayed Out" ("Disabled")
                      }
                      frame True {
                        n238 = case shown="True" w513 {
                          tunnel: [T2."Disabled and Grayed Out" ("Disabled") T2."Disabled and Grayed Out" ("Disabled")] -> w512
                          tunnel: [T2."Disabled and Grayed Out" ("Disabled") T2."Enabled" ("Disabled")] -> w511
                          tunnel: [T2."Enabled" ("Disabled") T2."Disabled and Grayed Out" ("Disabled")] -> w510
                          frame False {
                          }
                          frame True {
                          }
                        }
                        "authorized\nStatus" <- w514
                        "locked\nStatus" <- w513
                      }
                    }
                    n239 = property on="grant access" class="Bool"("DisabledEnum"=w500) -> ()  [unwired: 2 in, 2 out]
                    n240 = property on="Unlock" class="Bool"("DisabledEnum"=w499) -> ()  [unwired: 2 in, 2 out]
                    n241 = property on="Lock" class="Bool"("DisabledEnum"=w498) -> ()  [unwired: 2 in, 2 out]
                  }
                  event "device name (set)": Value Change {
                    n242 = event-data() -> ()  [unwired: 1 in, 1 out]
                    n243 = call "setDeviceName.vi"("name"="device name (set)", "connection ID"=w523) -> ("error out"=w522:errorcluster)  [unwired: 8 in, 1 out]
                  }
                  event "Lock": Value Change {
                    n244 = event-data() -> ()  [unwired: 1 in, 1 out]
                    n245 = call "Prompt User for Input2"() -> ("Password"=w524:string)  [unwired: 17 in, 2 out]
                    n246 = call "lock.vi"("password"=w524, "connection ID"=w526) -> ("error out"=w525:errorcluster)  [unwired: 8 in, 1 out]
                  }
                  event "Unlock": Value Change {
                    n247 = event-data() -> ()  [unwired: 1 in, 1 out]
                    n248 = call "Prompt User for Input3"() -> ("Password"=w527:string)  [unwired: 17 in, 2 out]
                    n249 = call "unlock.vi"("password"=w527, "connection ID"=w529) -> ("error out"=w528:errorcluster)  [unwired: 8 in, 1 out]
                  }
                  event "grant access": Value Change {
                    n250 = event-data() -> ()  [unwired: 1 in, 1 out]
                    n251 = call "Prompt User for Input4"() -> ("Password"=w530:string)  [unwired: 17 in, 2 out]
                    n252 = call "grantAccess.vi"("password"=w530, "connection ID"=w532) -> ("error out"=w531:errorcluster)  [unwired: 8 in, 1 out]
                  }
                  event "Reboot": Value Change {
                    n253 = event-data() -> ()  [unwired: 1 in, 1 out]
                    n254 = call "rebootSystem.vi"("connection ID"=w534) -> ("error out"=w533:errorcluster)  [unwired: 9 in, 1 out]
                  }
                  event "Factory Reset": Value Change {
                    n255 = event-data() -> ()  [unwired: 1 in, 1 out]
                    n256 = call "factoryReset.vi"("connection ID"=w536) -> ("error out"=w535:errorcluster)  [unwired: 9 in, 1 out]
                  }
                  event "Reset Error 8": Value Change {
                    n257 = event-data() -> ()  [unwired: 1 in, 1 out]
                    n258 = local write "Error 7"(FALSE ("Error 7")) -> ()
                    n259 = local write "Error Message 7"("" ("Error Message 9")) -> ()
                  }
                }
                n260 = Unbundle(w490) -> ("code"=w493:i32, "source"=w491:string)  [unwired: 1 out]
                n261 = Not Equal To 0?(x=w493) -> (x != 0?=w492:bool)
                n262 = case shown="True" w492 {
                  selector: w492 -> [_ w497]
                  tunnel: w491 -> [_ w496]
                  frame False {
                  }
                  frame True {
                    "Error Message 7" <- w496
                    "Error 7" <- w497
                  }
                }
              }
            }
          }
        }
        frame #2 {
          # "Exit / Disconnect"
          n263 = local write "stop"(FALSE ("stop")) -> ()
          n264 = call "close.vi"("connection ID"=w539) -> ()  [unwired: 6 in, 1 out]
        }
      }
    }
  }
